vi "UpdateSampleRate.vi"(3 "Task cluster in":T2={"Inbits"="Inbits", "Outbits"="Outbits", "Error Array"=[{"status"=FALSE, "code"=0, "source"=""}, {"status"=FALSE, "code"=0, "source"=""}, {"status"=FALSE, "code"=0, "source"=""}, {"status"=FALSE, "code"=0, "source"=""}, {"status"=FALSE, "code"=0, "source"=""}], "AO Array"=["AO 00-07", "AO 08-15", "AO 16-23"]}, 4 "Cue info":T1={"Duration (s)"=10.003, "Samps / sec"=10000.0, "Action Description"="send (2ms) and receive (10 s timeout. "}, 5 "milliseconds to wait":u32=100) -> (0 "Task cluster out":T2={"Inbits"="Inbits", "Outbits"="Outbits", "Error Array"=[{"status"=FALSE, "code"=0, "source"=""}, {"status"=FALSE, "code"=0, "source"=""}, {"status"=FALSE, "code"=0, "source"=""}, {"status"=FALSE, "code"=0, "source"=""}, {"status"=FALSE, "code"=0, "source"=""}], "AO Array"=["AO 00-07", "AO 08-15", "AO 16-23"]})   [LabVIEW 2018]
uses:
  Tasks.ctl
  <vilib>/DAQmx/configure/timing.llb/DAQmx Timing (Sample Clock).vi
panel:
  # "Tasks and errors"
  # "Tasks and errors"
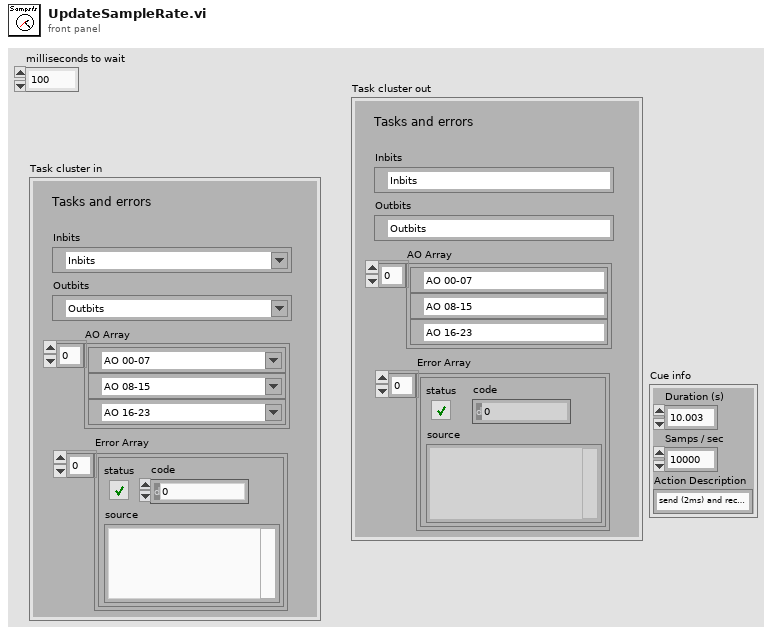
[diagram p1: front panel]
types:
  T1 = cluster{"Duration (s)":dbl, "Samps / sec":dbl, "Action Description":string}
  T2 = typedef "Tasks.ctl" = cluster{"Inbits":refnum<k21>, "Outbits":refnum<k21>, "Error Array":errorcluster[], "AO Array":refnum<k21>[]}
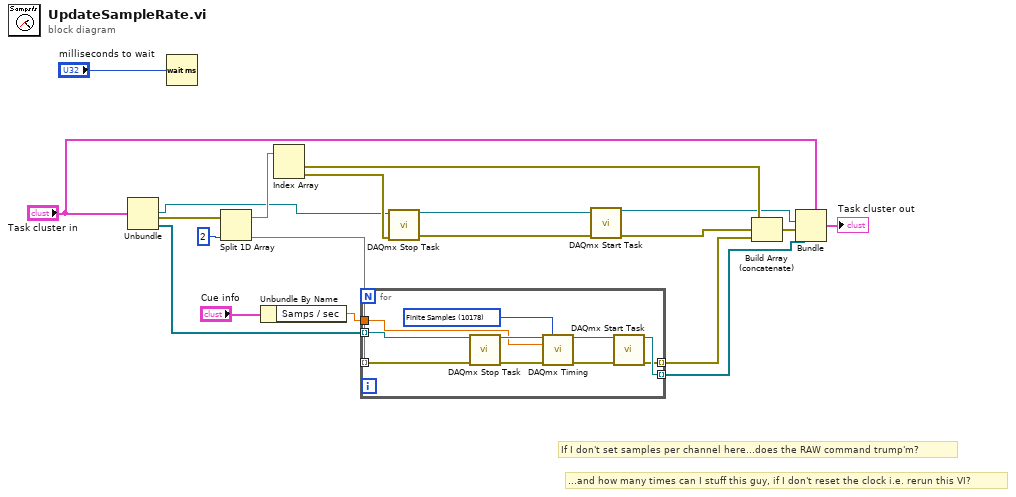
[diagram p0: block diagram]
diagram:
  # "...and how many times can I stuff this guy, if I don't reset the clock i.e. rerun this VI?"
  # "If I don't set samples per channel here...does the RAW command trump'm?"
  n1 = Unbundle("Task cluster in") -> ("Outbits"=w6:refnum<k21>, "Error Array"=w13:errorcluster[], "AO Array"=w12:refnum<k21>[])  [unwired: 1 out]
  n2 = Wait (ms)(milliseconds to wait="milliseconds to wait") -> ()  [unwired: 1 out]
  n3 = Split 1D Array(array=w13, index=2) -> (first subarray=w9:errorcluster[], second subarray=w15:errorcluster[])
  n4 = Unbundle By Name("Cue info") -> ("Samps / sec"=w3:dbl)
  n5 = Index Array(array=w9) -> (element #1=w8:errorcluster, element #2=w7:errorcluster)  [unwired: 2 in]
  n6 = for {
    tunnel: w3 -> [w28]
    tunnel: w12 -> [w25] mode=indexing
    tunnel: w15 -> [w24] mode=indexing
    tunnel: [w23] -> w17 mode=indexing
    tunnel: [w22] -> w18 mode=indexing
    w21 = 10178 items=["Finite Samples"=10178, "Continuous Samples"=10123, "Hardware Timed Single Point"=12522] ("sample mode")
    n7 = call <vilib>:"DAQmx Stop Task.vi"("task/channels in"=w25, "error in"=w24) -> ("task out"=w29:refnum<k21>, "error out"=w30:errorcluster)  [unwired: 12 in]
    n8 = call-poly <vilib>:"DAQmx Timing.vi"("task/channels in"=w29, "sample mode"=w21, "rate"=w28, "error in"=w30) -> ("task out"=w27:refnum<k21>, "error out"=w26:errorcluster)  [unwired: 10 in]
    n9 = call <vilib>:"DAQmx Start Task.vi"("task/channels in"=w27, "error in"=w26) -> ("task out"=w23:refnum<k21>, "error out"=w22:errorcluster)  [unwired: 12 in]
  }
  n10 = call <vilib>:"DAQmx Stop Task.vi"("task/channels in"=w6, "error in"=w7) -> ("task out"=w2:refnum<k21>, "error out"=w1:errorcluster)  [unwired: 12 in]
  n11 = call <vilib>:"DAQmx Start Task.vi"("task/channels in"=w2, "error in"=w1) -> ("task out"=w5:refnum<k21>, "error out"=w4:errorcluster)  [unwired: 12 in]
  n12 = Build Array (concatenate)(w8, w4, w18) -> (w19:errorcluster[])
  n13 = Bundle(cluster="Task cluster in", "Outbits"=w5, "Error Array"=w19, "AO Array"=w17) -> (→"Task cluster out":T2)  [unwired: 1 in]
